vi "ExSubNframeAccumCol.vi"(2 "error in (no error)":errorcluster, 3 "Number of Images":u32=1 min=1 step=1, 4 "Software accumulations":u32=1 min=1 step=1, 5 "Handle Cluster":T1) -> (0 "error out":errorcluster, 1 "Handle Cluster":T1)   [LabVIEW 2010]
panel:
  # "ExSubNframeAccumCol:\nThis is a sub VI that collects N frames from \nthe camera system. This assumes camera \nhas been setup and initialized and that the \nstart camera is done. this frame only stores \ndata when it has accumulated given amount, \nbut it does display intermediate sw accum\nvalues. It also assumes the camera has \ncircular buffer capabillities. This is not true for \nall cameras,  especially older cameras."
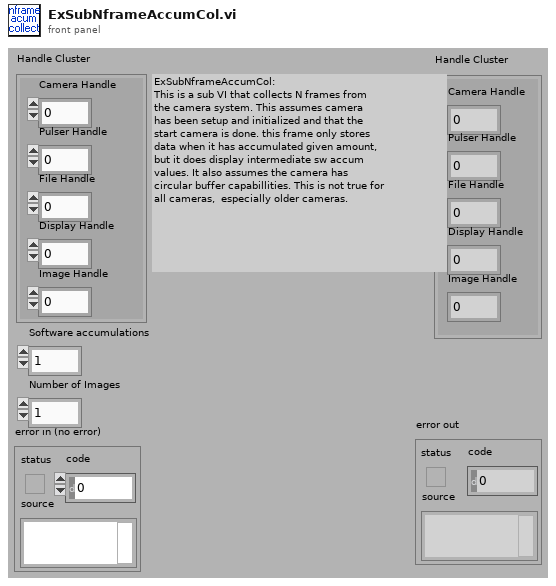
[diagram p1: front panel]
types:
  T1 = cluster{"Camera Handle":u32, "Pulser Handle":u32, "File Handle":u32, "Display Handle":u32, "Image Handle":u32}
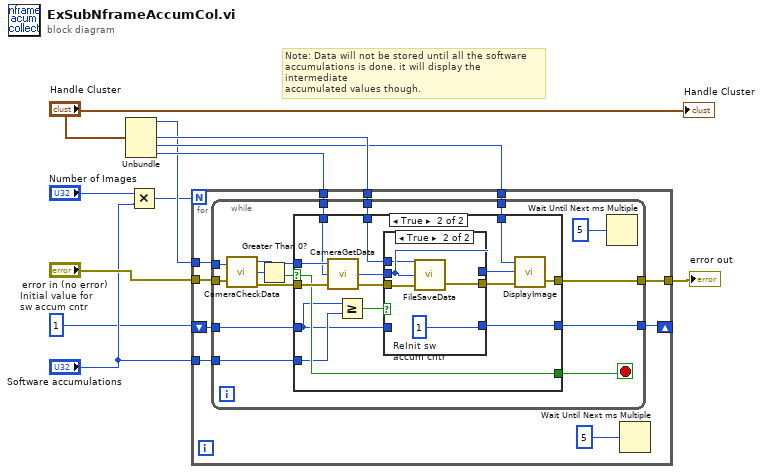
[diagram p0: block diagram]
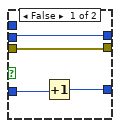
[diagram p3: hidden frame]
diagram:
  w1 = 1  # Initial value for  sw accum cntr
  # "Note: Data will not be stored until all the software \naccumulations is done. it will display the intermediate \naccumulated values though."
  n1 = Unbundle("Handle Cluster") -> ("Camera Handle"=w5:u32, "File Handle"=w11:u32, "Display Handle"=w10:u32, "Image Handle"=w9:u32)  [unwired: 1 out]
  n2 = Multiply(x="Number of Images", y="Software accumulations") -> (x*y=w3:u32)
  n3 = for {
    N: w3 -> [_]
    tunnel: w5 -> [w21]
    tunnel: w11 -> [w20]
    tunnel: w10 -> [w19]
    tunnel: w9 -> [w18]
    tunnel: "error in (no error)" -> [w17]
    tunnel: "Software accumulations" -> [w14]
    tunnel: [w15] -> w6
    shift-right: [w12] -> _
    shift-left: w1 -> [w13]
    n4 = while {
      tunnel: w17 -> [w35]
      tunnel: w21 -> [w34]
      tunnel: [w29] -> w15
      tunnel: w20 -> [w28]
      tunnel: w19 -> [w27]
      tunnel: w18 -> [w26]
      tunnel: w14 -> [w24]
      tunnel: w13 -> [w23]
      tunnel: [w22] -> w12
      stop <- w30 stop-if-true
      n5 = call <userlib>:"CameraCheckData.vi"("Camera Handle"=w34, "error in"=w35) -> ("Camera Handle"=w32:u32, "Number Of Frames Available"=w36:i32, "error out"=w31:errorcluster)
      n6 = Greater Than 0?(x=w36) -> (x > 0?=w33:bool)
      n7 = case shown="True" w33 {
        selector: w33 -> [w38 w52]
        tunnel: w32 -> [_ w54]
        tunnel: w31 -> [w39 w53]
        tunnel: [w38 w52] -> w30
        tunnel: [w39 w51] -> w29
        tunnel: w28 -> [_ w43]
        tunnel: w27 -> [_ w50]
        tunnel: w26 -> [_ w49]
        tunnel: w24 -> [_ w42]
        tunnel: w23 -> [w37 w41]
        tunnel: [w37 w40] -> w22
        frame False {
        }
        frame True {
          n8 = call <userlib>:"CameraGetData.vi"("error in"=w53, "Data Handle"=w49, "Camera Handle"=w54) -> ("error out"=w47:errorcluster, "Data Handle"=w46:u32)  [unwired: 1 out]
          n9 = Greater Or Equal?(x=w41, y=w42) -> (x >= y?=w48:bool)
          n10 = case shown="True" w48 {
            tunnel: w47 -> [w58 w63]
            tunnel: w46 -> [w57 w61]
            tunnel: [w58 w62] -> w45
            tunnel: [w57 w61] -> w44
            tunnel: w43 -> [_ w60]
            tunnel: w41 -> [w56 _]
            tunnel: [w55 w59] -> w40
            frame False {
              n11 = Increment(x=w56) -> (x+1=w55:i32)
            }
            frame True {
              w59 = 1  # ReInit sw  accum cntr
              n12 = call <userlib>:"FileSaveData.vi"("error in"=w63, "Image Handle"=w61, "File Handle"=w60) -> ("error out"=w62:errorcluster)  [unwired: 1 out]
            }
          }
          n13 = call <userlib>:"DisplayImage.vi"("error in"=w45, "Image Handle"=w44, "Display Handle"=w50) -> ("error out"=w51:errorcluster)  [unwired: 1 in, 1 out]
        }
      }
      n14 = Wait Until Next ms Multiple(millisecond multiple=u32 5) -> ()  [unwired: 1 out]
    }
    n15 = Wait Until Next ms Multiple(millisecond multiple=u32 5) -> ()  [unwired: 1 out]
  }
  "error out" <- w6
  "Handle Cluster" <- "Handle Cluster"
